vi "final_project.vi"() -> ()   [LabVIEW 2019]
uses:
  ProgramStatusController.ctl
  States.ctl
  CMDs.ctl
  <vilib>/Utility/file.llb/Write Delimited Spreadsheet (string).vi
panel:
  in  "Record file path (dialog if empty)":path
  out "Status String":string
  in  "Measure&Log All":bool
  in  "MeasureGP":bool
  in  "MeasureGV":bool
  in  "MeasureGT":bool
  in  "MeasureWT":bool
  in  "MeasureFT":bool
  out "Greenhouse PAR:":u16 format="%#.0f"
  out "Greenhouse VPD (kPa):":dbl format="%.3g"
  out "Greenhouse Temperature:":dbl format="%.1g"
  out "Wine Cellar Temperature:":dbl format="%.1f"
  out "Fridge Temperature:":dbl format="%.1f"
  in  "Serial Communication Port:":refnum<visa-resource-name>="COM1"
  # "Measurements are made and logged automatically\nevery 5 minutes.\n\nFor manual logging, press the \"Measure & Log All\"\nbutton above.\n\nFor an individual measurement, without logging press the corresponding \"Measure\" button above."
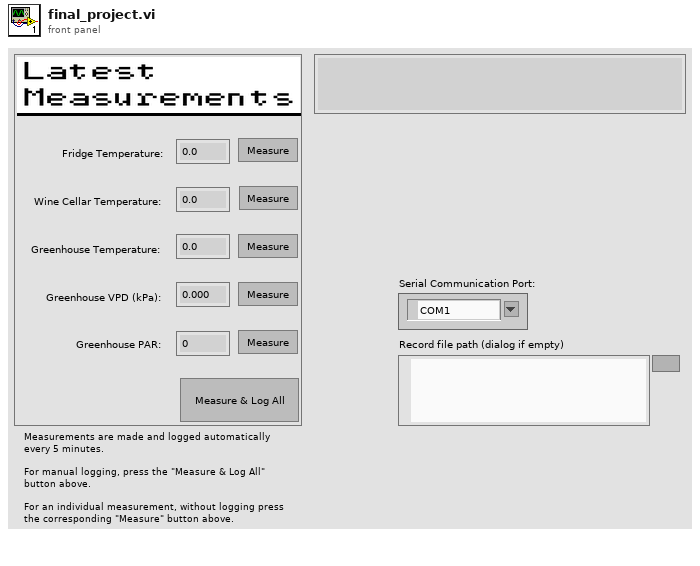
[diagram p1: front panel]
types:
  T1 = typedef "ProgramStatusController.ctl" = cluster{"LogTimer":u64, "StatusMsgTimer":u64, "State":T2, "Measure CDM":T3}
  T2 = typedef "States.ctl" = enum16{"WaitForAction", "MeasureAndLog", "PerformMeasure"}
  T3 = typedef "CMDs.ctl" = enum16{"UNK", "FridgeTemp", "WineCellarTemp", "GreenhouseTemp", "GreenhouseVPD", "GreenhousePAR"}
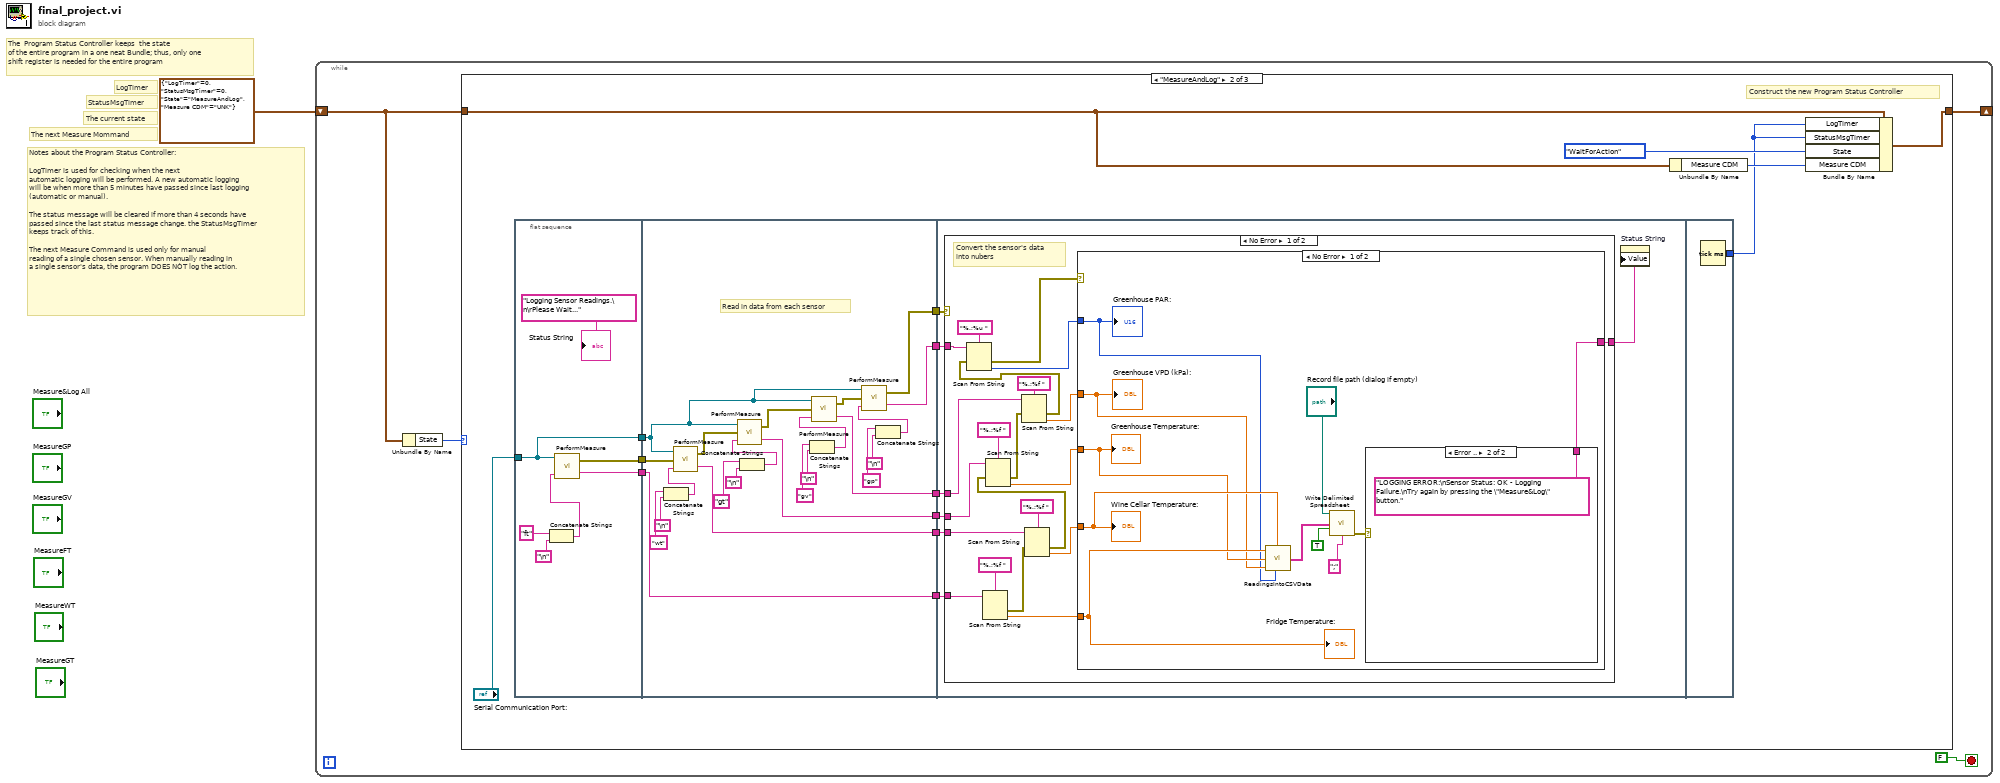
[diagram p0: block diagram]
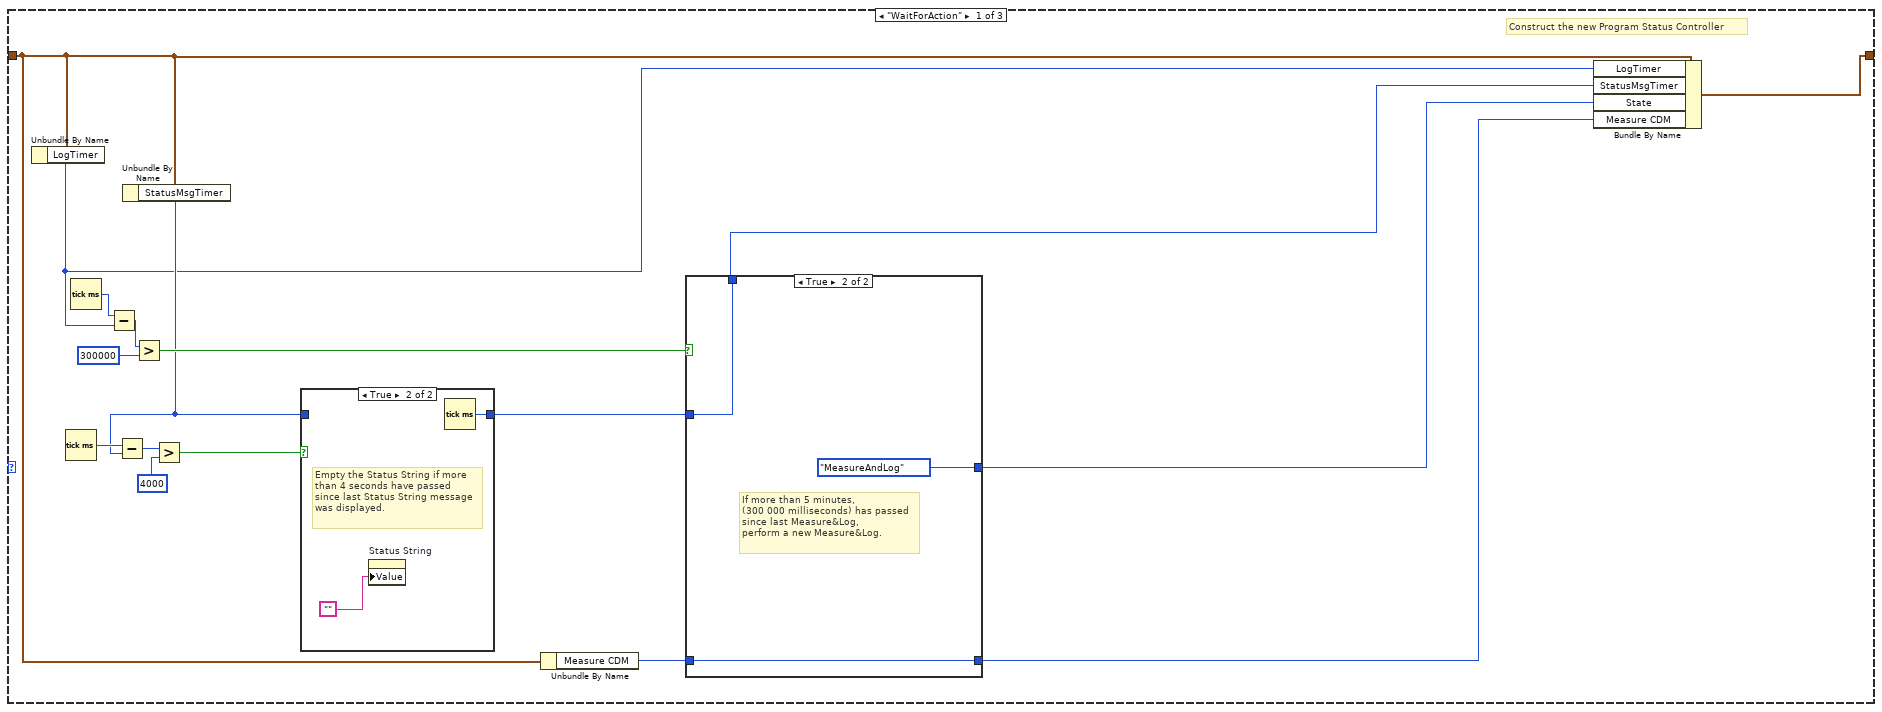
[diagram p2: hidden frame]
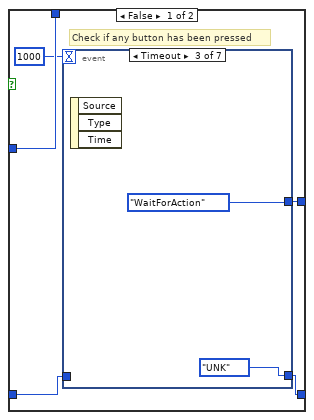
[diagram p4: hidden frame]
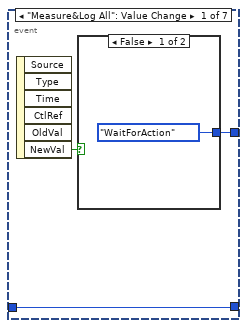
[diagram p5: hidden frame]
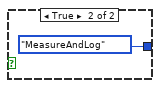
[diagram p6: hidden frame]
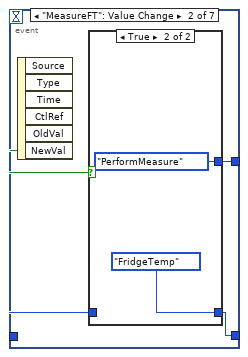
[diagram p7: hidden frame]
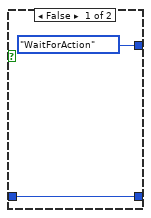
[diagram p8: hidden frame]
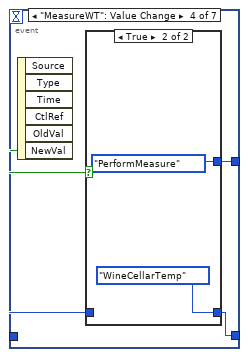
[diagram p9: hidden frame]
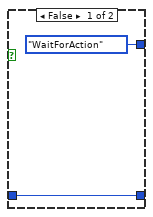
[diagram p10: hidden frame]
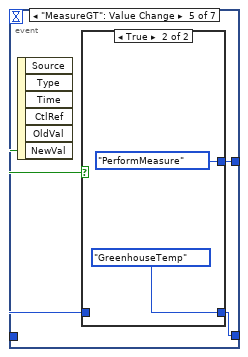
[diagram p11: hidden frame]
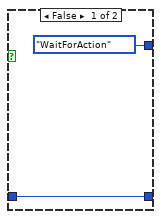
[diagram p12: hidden frame]
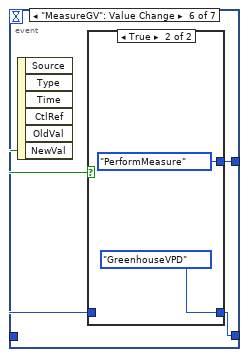
[diagram p13: hidden frame]
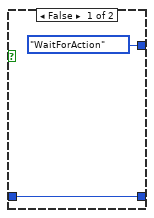
[diagram p14: hidden frame]
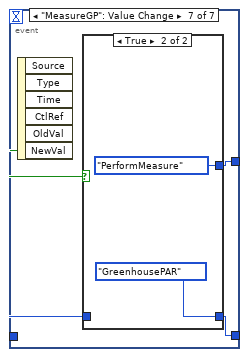
[diagram p15: hidden frame]
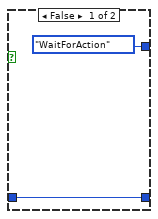
[diagram p16: hidden frame]
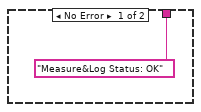
[diagram p17: hidden frame]
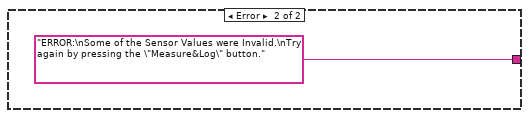
[diagram p18: hidden frame]
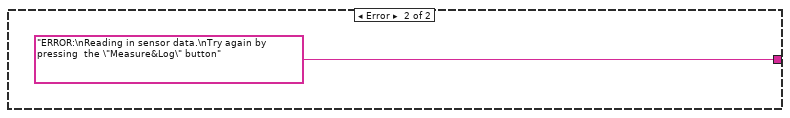
[diagram p19: hidden frame]
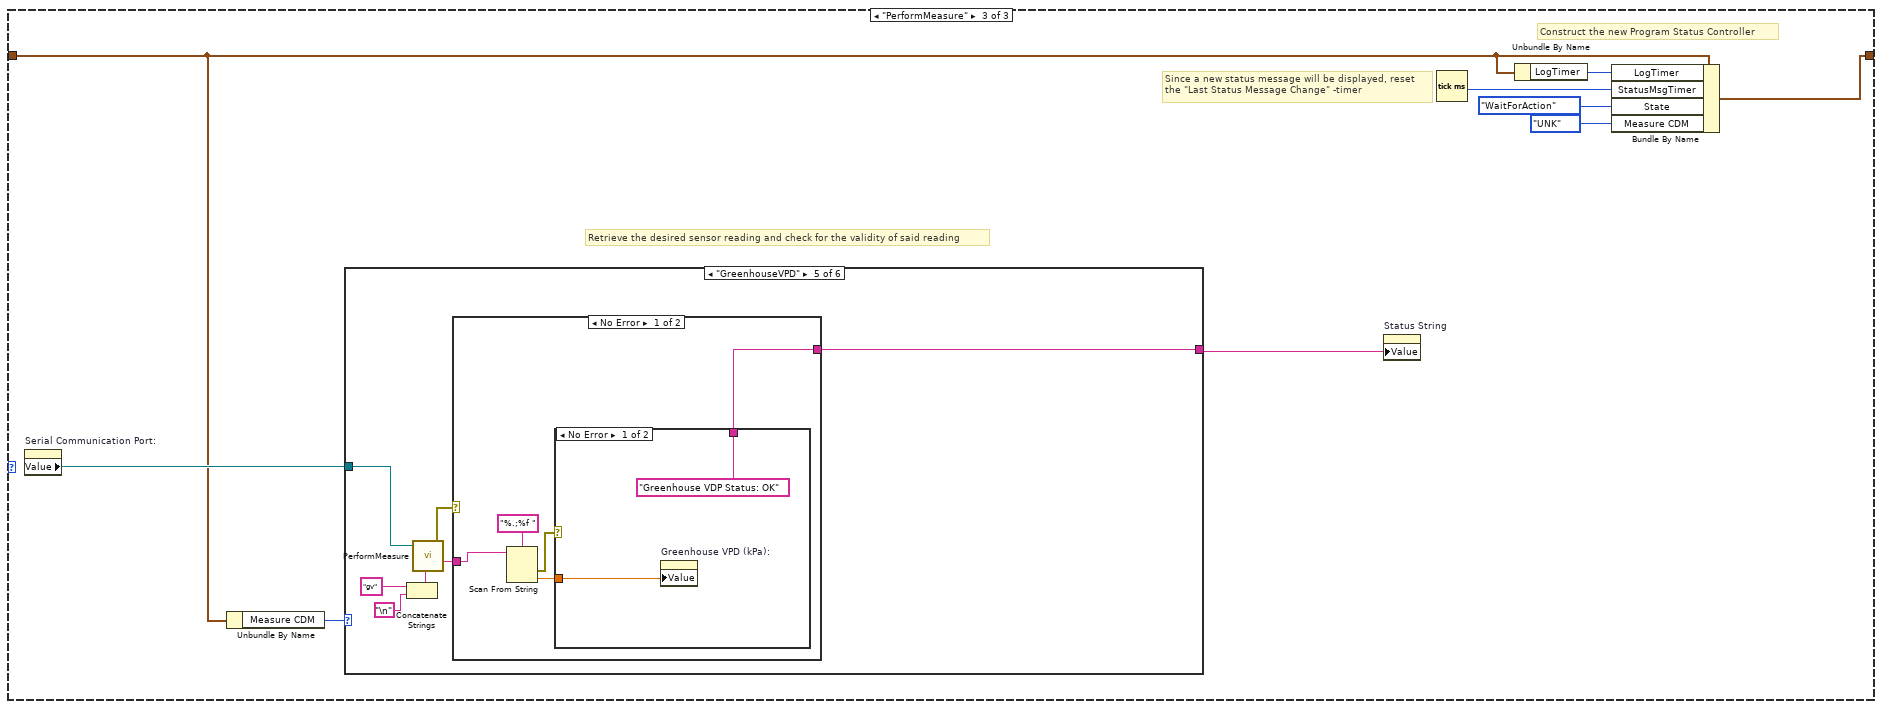
[diagram p20: hidden frame]
diagram:
  # "Notes about the Program Status Controller:\n\nLogTimer is used for checking when the next\nautomatic logging will be performed. A new automatic logging\nwill be when more than 5 minutes have passed since last logging\n(automatic or manual).\n\nThe status message will be cleared if more than 4 seconds have\npassed since the last status message change. the StatusMsgTimer\nkeeps track of this.\n\nThe next Measure Command is used only for manual\nreading of a single chosen sensor. When manually reading in\na single sensor's data, the program DOES NÒT log the action."
  # "The  Program Status Controller keeps  the state\nof the entire program in a one neat Bundle; thus, only one\nshift register is needed for the entire program"
  # "The next Measure Mommand"
  # "The current state"
  # "StatusMsgTimer"
  # "LogTimer"
  n1 = while {
    shift-right: [w4] -> _
    shift-left: T1 {"LogTimer"=0, "StatusMsgTimer"=0, "State"=enum."MeasureAndLog", "Measure CDM"=enum."UNK"} -> [w2]
    stop <- FALSE stop-if-true
    n2 = Unbundle By Name(w2) -> ("State"=w3:T2)
    n3 = case shown="\"MeasureAndLog\"" w3 {
      tunnel: [w13 w85 w172] -> w4
      tunnel: w2 -> [w6 w83 w171]
      frame "WaitForAction" {
        # "Construct the new Program Status Controller"
        n4 = Unbundle By Name(w6) -> ("LogTimer"=w8:u64)
        n5 = Tick Count (ms)() -> (millisecond timer value=w18:u32)
        n6 = Tick Count (ms)() -> (millisecond timer value=w19:u32)
        n7 = Subtract(x=w19, y=w8) -> (x-y=w22:u64)
        n8 = Unbundle By Name(w6) -> ("StatusMsgTimer"=w9:u64)
        n9 = Subtract(x=w18, y=w9) -> (x-y=w17:u64)
        n10 = Greater?(x=w22, y=300000) -> (0:w20:bool)
        n11 = Greater?(x=w17, y=4000) -> (0:w15:bool)
        n12 = case shown="True" w15 {
          tunnel: w9 -> [w23 _]
          tunnel: [w23 w25] -> w14
          frame False {
          }
          frame True {
            # "Empty the Status String if more\nthan 4 seconds have passed\nsince last Status String message\nwas displayed."
            n13 = property on="Status String" class="Str"("Value"="") -> ()  [unwired: 2 in, 2 out]
            n14 = Tick Count (ms)() -> (millisecond timer value=w25:u32)
          }
        }
        n15 = Unbundle By Name(w6) -> ("Measure CDM"=w7:T3)
        n16 = case shown="True" w20 {
          tunnel: w7 -> [w30 w80]
          tunnel: [w29 w80] -> w10
          tunnel: [w28 States."MeasureAndLog"] -> w11
          tunnel: w14 -> [w27 w78]
          tunnel: [w27 w78] -> w12
          frame False {
            # "Check if any button has been pressed"
            n17 = event shown="[2] Timeout" {
              selector: _ -> [_ _ _ _ _ _ _]
              dyn-events: _ -> [_ _ _ _ _ _ _]
              timeout: 1000 -> [_ _ _ _ _ _ _]
              tunnel: w30 -> [w32 w38 _ w48 w56 w63 w73]
              tunnel: [w32 w37 CMDs."UNK" ("Enum") w49 w55 w64 w72] -> w29
              tunnel: [w31 w36 States."WaitForAction" w47 w57 w65 w71] -> w28
              event "Measure&Log All": Value Change {
                n18 = event-data() -> ("NewVal"=w33:bool)  [unwired: 1 in, 5 out]
                n19 = case shown="False" w33 {
                  tunnel: [States."WaitForAction" States."MeasureAndLog"] -> w31
                  frame False {
                  }
                  frame True {
                  }
                }
              }
              event "MeasureFT": Value Change {
                n20 = event-data() -> ("NewVal"=w39:bool)  [unwired: 1 in, 5 out]
                n21 = case shown="True" w39 {
                  tunnel: w38 -> [w41 _]
                  tunnel: [w41 CMDs."FridgeTemp"] -> w37
                  tunnel: [States."WaitForAction" States."PerformMeasure"] -> w36
                  frame False {
                  }
                  frame True {
                  }
                }
              }
              event Timeout {
                n22 = event-data() -> ()  [unwired: 1 in, 3 out]
              }
              event "MeasureWT": Value Change {
                n23 = event-data() -> ("NewVal"=w46:bool)  [unwired: 1 in, 5 out]
                n24 = case shown="True" w46 {
                  tunnel: w48 -> [w51 _]
                  tunnel: [w51 CMDs."WineCellarTemp"] -> w49
                  tunnel: [States."WaitForAction" States."PerformMeasure"] -> w47
                  frame False {
                  }
                  frame True {
                  }
                }
              }
              event "MeasureGT": Value Change {
                n25 = event-data() -> ("NewVal"=w54:bool)  [unwired: 1 in, 5 out]
                n26 = case shown="True" w54 {
                  tunnel: w56 -> [w59 _]
                  tunnel: [w59 CMDs."GreenhouseTemp"] -> w55
                  tunnel: [States."WaitForAction" States."PerformMeasure"] -> w57
                  frame False {
                  }
                  frame True {
                  }
                }
              }
              event "MeasureGV": Value Change {
                n27 = event-data() -> ("NewVal"=w62:bool)  [unwired: 1 in, 5 out]
                n28 = case shown="True" w62 {
                  tunnel: w63 -> [w67 _]
                  tunnel: [w67 CMDs."GreenhouseVPD"] -> w64
                  tunnel: [States."WaitForAction" States."PerformMeasure"] -> w65
                  frame False {
                  }
                  frame True {
                  }
                }
              }
              event "MeasureGP": Value Change {
                n29 = event-data() -> ("NewVal"=w70:bool)  [unwired: 1 in, 5 out]
                n30 = case shown="True" w70 {
                  tunnel: w73 -> [w75 _]
                  tunnel: [w75 CMDs."GreenhousePAR"] -> w72
                  tunnel: [States."WaitForAction" States."PerformMeasure"] -> w71
                  frame False {
                  }
                  frame True {
                  }
                }
              }
            }
          }
          frame True {
            # "If more than 5 minutes,\n(300 000 milliseconds) has passed\nsince last Measure&Log,\nperform a new Measure&Log."
          }
        }
        n31 = Bundle By Name(cluster=w6, "LogTimer"=w8, "StatusMsgTimer"=w12, "State"=w11, "Measure CDM"=w10) -> (w13:T1)
      }
      frame "MeasureAndLog" {
        # "Construct the new Program Status Controller"
        n32 = flat-sequence {
          tunnel: [w98] -> w95
          tunnel: [w97] -> w94
          tunnel: "Serial Communication Port:" -> [w96]
          tunnel: [w96] -> w91
          tunnel: w95 -> [w125]
          tunnel: w94 -> [w124]
          tunnel: [w124] -> w93
          tunnel: w91 -> [w108]
          tunnel: [w120] -> w90
          tunnel: [w115] -> w89
          tunnel: [w110] -> w88
          tunnel: [w104] -> w87
          tunnel: [w103] -> w86
          tunnel: w93 -> [w126]
          tunnel: w90 -> [w127]
          tunnel: w89 -> [w128]
          tunnel: w88 -> [w129]
          tunnel: w87 -> [w130]
          tunnel: w86 -> [w132]
          tunnel: [w169] -> w81
          frame #0 {
            n33 = Concatenate Strings("ft", "\n") -> (w99:string)
            n34 = call "PerformMeasure.vi"("Command"=w99, "Serial Communication Port:"=w96) -> ("Response"=w97:string, "error out"=w98:errorcluster)  [unwired: 1 in]
            "Status String" <- "Logging Sensor Readings.\n\rPlease Wait..."
          }
          frame #1 {
            # "Read in data from each sensor"
            n35 = Concatenate Strings("wt", "\n") -> (w121:string)
            n36 = call "PerformMeasure.vi"("Command"=w121, "error in"=w125, "Serial Communication Port:"=w108) -> ("Response"=w120:string, "error out"=w116:errorcluster)
            n37 = Concatenate Strings("gt", "\n") -> (w117:string)
            n38 = call "PerformMeasure.vi"("Command"=w117, "error in"=w116, "Serial Communication Port:"=w108) -> ("Response"=w115:string, "error out"=w114:errorcluster)
            n39 = Concatenate Strings("gv", "\n") -> (w111:string)
            n40 = call "PerformMeasure.vi"("Command"=w111, "error in"=w114, "Serial Communication Port:"=w108) -> ("Response"=w110:string, "error out"=w109:errorcluster)
            n41 = Concatenate Strings("gp", "\n") -> (w105:string)
            n42 = call "PerformMeasure.vi"("Command"=w105, "error in"=w109, "Serial Communication Port:"=w108) -> ("Response"=w104:string, "error out"=w103:errorcluster)
          }
          frame #2 {
            n43 = case shown="No Error" w132 {
              tunnel: [w133 "ERROR:\nReading in sensor data.\nTry again by pressing  the \"Measure&Log\" button"] -> w131
              tunnel: w130 -> [w134 _]
              tunnel: w129 -> [w135 _]
              tunnel: w128 -> [w136 _]
              tunnel: w127 -> [w137 _]
              tunnel: w126 -> [w138 _]
              frame No Error {
                # "Convert the sensor's data \ninto nubers"
                n44 = Scan From String(format string="%.;%f ", input string=w138) -> (error out=w143:errorcluster, output 1=w144:dbl)  [unwired: 3 in, 2 out]
                n45 = Scan From String(format string="%.;%f ", input string=w137, error in=w143) -> (error out=w142:errorcluster, output 1=w145:dbl)  [unwired: 2 in, 2 out]
                n46 = Scan From String(format string="%.;%f ", input string=w136, error in=w142) -> (error out=w141:errorcluster, output 1=w146:dbl)  [unwired: 2 in, 2 out]
                n47 = Scan From String(format string="%.;%f ", input string=w135, error in=w141) -> (error out=w140:errorcluster, output 1=w147:dbl)  [unwired: 2 in, 2 out]
                n48 = Scan From String(format string="%.;%u ", input string=w134, error in=w140) -> (error out=w139:errorcluster, output 1=w148:u32)  [unwired: 2 in, 2 out]
                n49 = case shown="No Error" w139 {
                  tunnel: w148 -> [w154 _]
                  tunnel: w147 -> [w155 _]
                  tunnel: w146 -> [w156 _]
                  tunnel: w145 -> [w158 _]
                  tunnel: w144 -> [w157 _]
                  tunnel: [w160 "ERROR:\nSome of the Sensor Values were Invalid.\nTry again by pressing the \"Measure&Log\" button."] -> w133
                  frame No Error {
                    n50 = call "ReadingsIntoCSVData.vi"("Fridge Temoerature"=w157, "Wine Cellar Temperature"=w158, "Greenhouse Temperature"=w156, "Greenhouse VPD"=w155, "Greenhouse PAR"=w154) -> ("Array"=w159:string[])
                    n51 = call-poly <vilib>:"Write Delimited Spreadsheet.vi"("file path (dialog if empty)"="Record file path (dialog if empty)", "1D data"=w159, "append to file? (new file:F)"=TRUE, "delimiter (\\t)"=";") -> ("error out"=w161:errorcluster)  [unwired: 10 in, 1 out]
                    n52 = case shown="Error .." w161 {
                      tunnel: ["Measure&Log Status: OK" "LOGGING ERROR:\nSensor Status: OK - Logging Failure.\nTry again by pressing the \"Measure&Log\" button."] -> w160
                      frame No Error {
                      }
                      frame Error {
                      }
                    }
                    "Greenhouse PAR:" <- w154
                    "Greenhouse VPD (kPa):" <- w155
                    "Fridge Temperature:" <- w157
                    "Greenhouse Temperature:" <- w156
                    "Wine Cellar Temperature:" <- w158
                  }
                  frame Error {
                  }
                }
              }
              frame Error {
              }
            }
            n53 = property on="Status String" class="Str"("Value"=w131) -> ()  [unwired: 2 in, 2 out]
          }
          frame #3 {
            n54 = Tick Count (ms)() -> (millisecond timer value=w169:u32)
          }
        }
        n55 = Unbundle By Name(w83) -> ("Measure CDM"=w84:T3)
        n56 = Bundle By Name(cluster=w83, "LogTimer"=w81, "StatusMsgTimer"=w81, "State"=States."WaitForAction", "Measure CDM"=w84) -> (w85:T1)
      }
      frame "PerformMeasure" {
        # "Construct the new Program Status Controller"
        # "Since a new status message will be displayed, reset\nthe \"Last Status Message Change\" -timer"
        # "Retrieve the desired sensor reading and check for the validity of said reading"
        n57 = property on="Serial Communication Port:" class="VISAName"() -> ("Value"=w177:refnum<visa-resource-name>)  [unwired: 2 in, 2 out]
        n58 = Unbundle By Name(w171) -> ("Measure CDM"=w170:T3)
        n59 = case shown="\"GreenhouseVPD\"" w170 {
          tunnel: ["ERROR:\nUnknown Measurement" w186 w202 w215 w231 w250] -> w178
          tunnel: w177 -> [_ w184 w199 w218 w234 w247]
          frame "UNK" {
          }
          frame "FridgeTemp" {
            n60 = Concatenate Strings("ft", "\n") -> (w180:string)
            n61 = call "PerformMeasure.vi"("Command"=w180, "Serial Communication Port:"=w184) -> ("Response"=w183:string, "error out"=w185:errorcluster)  [unwired: 1 in]
            n62 = case shown="Error" w185 {
              tunnel: [w188 "ERROR:\nreading in Fridge Temperature "] -> w186
              tunnel: w183 -> [w191 _]
              frame No Error {
                n63 = Scan From String(format string="%.;%f ", input string=w191) -> (error out=w189:errorcluster, output 1=w187:dbl)  [unwired: 3 in, 2 out]
                n64 = case shown="No Error" w189 {
                  tunnel: w187 -> [w193 _]
                  tunnel: ["Fridge Temperature Status: OK" "ERROR:\nInvalid Fridge Temperature value"] -> w188
                  frame No Error {
                    n65 = property on="Fridge Temperature:" class="DigNum (strict)"("Value"=w193) -> ()  [unwired: 2 in, 2 out]
                  }
                  frame Error {
                  }
                }
              }
              frame Error {
              }
            }
          }
          frame "WineCellarTemp" {
            n66 = Concatenate Strings("wt", "\n") -> (w198:string)
            n67 = call "PerformMeasure.vi"("Command"=w198, "Serial Communication Port:"=w199) -> ("Response"=w201:string, "error out"=w200:errorcluster)  [unwired: 1 in]
            n68 = case shown="No Error" w200 {
              tunnel: [w203 "ERROR:\nreading in Wine Cellar Temperature"] -> w202
              tunnel: w201 -> [w206 _]
              frame No Error {
                n69 = Scan From String(format string="%.;%f ", input string=w206) -> (error out=w205:errorcluster, output 1=w204:dbl)  [unwired: 3 in, 2 out]
                n70 = case shown="No Error" w205 {
                  tunnel: w204 -> [w209 _]
                  tunnel: ["Wince Cellar Temperature Status: OK" "ERROR:\nInvalid Wine Cellar Temperature Value"] -> w203
                  frame No Error {
                    n71 = property on="Wine Cellar Temperature:" class="DigNum (strict)"("Value"=w209) -> ()  [unwired: 2 in, 2 out]
                  }
                  frame Error {
                  }
                }
              }
              frame Error {
              }
            }
          }
          frame "GreenhouseTemp" {
            n72 = Concatenate Strings("gt", "\n") -> (w214:string)
            n73 = call "PerformMeasure.vi"("Command"=w214, "Serial Communication Port:"=w218) -> ("Response"=w216:string, "error out"=w217:errorcluster)  [unwired: 1 in]
            n74 = case shown="No Error" w217 {
              tunnel: w216 -> [w223 _]
              tunnel: [w219 "ERROR:\nreading in Greenhouse Temperature"] -> w215
              frame No Error {
                n75 = Scan From String(format string="%.;%f ", input string=w223) -> (error out=w221:errorcluster, output 1=w220:dbl)  [unwired: 3 in, 2 out]
                n76 = case shown="No Error" w221 {
                  tunnel: w220 -> [w225 _]
                  tunnel: ["Greenhouse Temperature Status: OK" "ERROR:\nIllegal Greenhouse Temperature Value"] -> w219
                  frame No Error {
                    n77 = property on="Greenhouse Temperature:" class="DigNum (strict)"("Value"=w225) -> ()  [unwired: 2 in, 2 out]
                  }
                  frame Error {
                  }
                }
              }
              frame Error {
              }
            }
          }
          frame "GreenhouseVPD" {
            n78 = Concatenate Strings("gv", "\n") -> (w230:string)
            n79 = call "PerformMeasure.vi"("Command"=w230, "Serial Communication Port:"=w234) -> ("Response"=w232:string, "error out"=w233:errorcluster)  [unwired: 1 in]
            n80 = case shown="No Error" w233 {
              tunnel: w232 -> [w238 _]
              tunnel: [w236 "ERROR:\nreading in greenhouse VPD"] -> w231
              frame No Error {
                n81 = Scan From String(format string="%.;%f ", input string=w238) -> (error out=w237:errorcluster, output 1=w235:dbl)  [unwired: 3 in, 2 out]
                n82 = case shown="No Error" w237 {
                  tunnel: ["Greenhouse VDP Status: OK" "ERROR:\nInvalid Greenhouse VDP value"] -> w236
                  tunnel: w235 -> [w240 _]
                  frame No Error {
                    n83 = property on="Greenhouse VPD (kPa):" class="DigNum (strict)"("Value"=w240) -> ()  [unwired: 2 in, 2 out]
                  }
                  frame Error {
                  }
                }
              }
              frame Error {
              }
            }
          }
          frame "GreenhousePAR" {
            n84 = Concatenate Strings("gp", "\n") -> (w246:string)
            n85 = call "PerformMeasure.vi"("Command"=w246, "Serial Communication Port:"=w247) -> ("Response"=w248:string, "error out"=w249:errorcluster)  [unwired: 1 in]
            n86 = case shown="No Error" w249 {
              tunnel: [w251 "ERROR:\nreading in greenhouse PAR status"] -> w250
              tunnel: w248 -> [w255 _]
              frame No Error {
                n87 = Scan From String(format string="%.;%u ", input string=w255) -> (error out=w253:errorcluster, output 1=w252:u32)  [unwired: 3 in, 2 out]
                n88 = case shown="No Error" w253 {
                  tunnel: w252 -> [w257 _]
                  tunnel: ["Greenhouse PAR Status: OK" "ERROR:\nInvalid Greenhouse PAR value"] -> w251
                  frame No Error {
                    n89 = property on="Greenhouse PAR:" class="DigNum (strict)"("Value"=w257) -> ()  [unwired: 2 in, 2 out]
                  }
                  frame Error {
                  }
                }
              }
              frame Error {
              }
            }
          }
        }
        n90 = property on="Status String" class="Str"("Value"=w178) -> ()  [unwired: 2 in, 2 out]
        n91 = Tick Count (ms)() -> (millisecond timer value=w176:u32)
        n92 = Unbundle By Name(w171) -> ("LogTimer"=w173:u64)
        n93 = Bundle By Name(cluster=w171, "LogTimer"=w173, "StatusMsgTimer"=w176, "State"=States."WaitForAction", "Measure CDM"=CMDs."UNK") -> (w172:T1)
      }
    }
  }
